vi "Init lib MPSSE.vi"(11 "error in (no error)":errorcluster) -> (15 "error out":errorcluster)   [LabVIEW 2017, in "libMPSSE.lvlib"]
doc: "FTDI_API void Init_libMPSSE(void);"
uses:
  libMPSSE.lvlib
  libMPSSE-SPI-LabVIEW-master/libMPSSE.dll
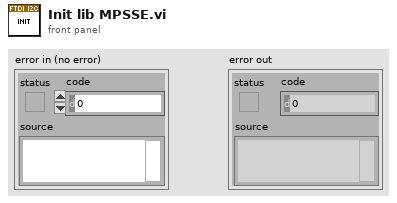
[diagram p1: front panel]
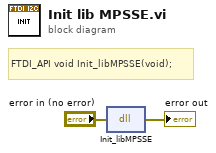
[diagram p0: block diagram]
diagram:
  # "FTDI_API void Init_libMPSSE(void);"
  n1 = dll-call lib="\\\\Mac\\Home/Desktop/libMPSSE-SPI-LabVIEW-master/libMPSSE.dll" fn="Init_libMPSSE"(error in="error in (no error)") -> (error out=→"error out":errorcluster)  [unwired: 3 in, 1 out]
